vi "Set Adapter.vi"(8 "error in (no error)":errorcluster, 10 "I Authentication Provider":refnum<class "I Authentication Provider.lvclass">, 11 "Authentication Service in":refnum<class "Authentication Service.lvclass">) -> (0 "error out":errorcluster, 3 "Authentication Service out":refnum<class "Authentication Service.lvclass">)   [LabVIEW 2026, in "Authentication Service.lvclass"]
uses:
  Authentication Service.lvclass
  Authentication Service.lvclass/Authentication Service.ctl
  Interfaces/I Authentication Provider/I Authentication Provider.lvclass
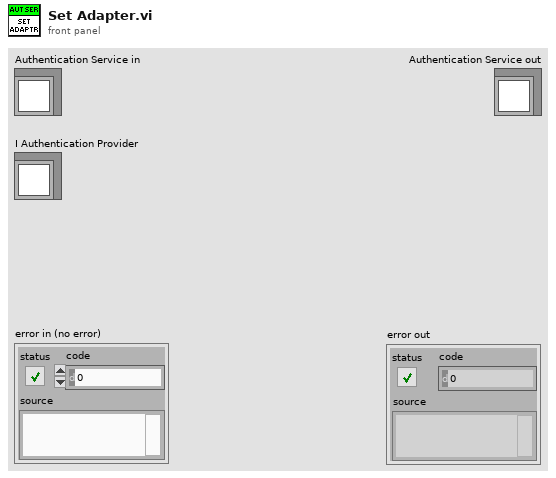
[diagram p1: front panel]
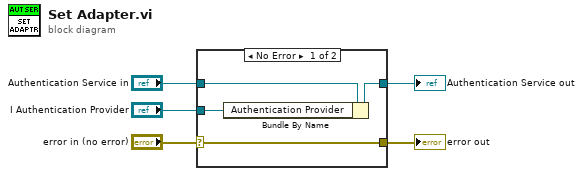
[diagram p0: block diagram]
diagram:
  n1 = case shown="No Error" "error in (no error)" {
    selector: "error in (no error)" -> [w9 w10]
    tunnel: [w9 w10] -> w4
    tunnel: [w6 w11] -> w3
    tunnel: "Authentication Service in" -> [w8 w11]
    tunnel: "I Authentication Provider" -> [w7 _]
    frame No Error {
      n2 = Bundle By Name(cluster=w8, "Authentication Provider"=w7) -> (w6:refnum<class "Authentication Service.lvclass">)
    }
    frame Error {
    }
  }
  "Authentication Service out" <- w3
  "error out" <- w4
